vi "Host Trigger Detect.vi"(11 "Software Trigger from Host":bool) -> (2 "Host Rising Edge Detect":bool)   [LabVIEW 2012]
uses:
  <instrlib>/FlexRIO/Libraries/Helper VIs/NI FlexRIO Helper VIs.lvlib
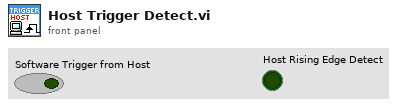
[diagram p1: front panel]
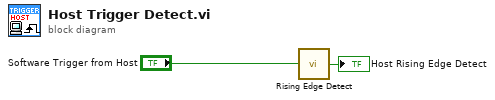
[diagram p0: block diagram]
diagram:
  n1 = call <instrlib>:"Rising Edge Detect.vi"("signal"="Software Trigger from Host") -> ("edge detected"=→"Host Rising Edge Detect":bool)  [unwired: 14 in]
